vi "Normalize String.vi"(0 "String":string) -> (2 "Normalized String":string)   [LabVIEW 2013, in "JUnit XML.lvlib"]
doc: "Normalizes a string accordign to the XML specification."
uses:
  JUnit XML.lvlib
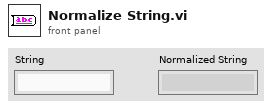
[diagram p1: front panel]
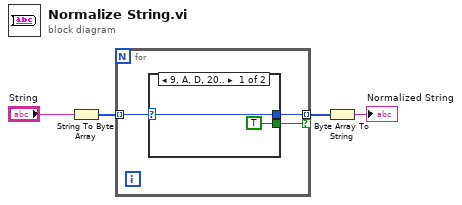
[diagram p0: block diagram]
diagram:
  n1 = String To Byte Array(string="String") -> (unsigned byte array=w3:u8[])
  n2 = for {
    tunnel: w3 -> [w7] mode=indexing
    tunnel: [w6] -> w2 mode=indexing if=w5
    n3 = case shown="9, A, D, 20.." w7 {
      selector: w7 -> [w8 _]
      tunnel: [w8 _] -> w6
      tunnel: [TRUE _] -> w5
      frame 9, 10, 13, 32.. {
      }
      frame Default {
      }
    }
  }
  n4 = Byte Array To String(unsigned byte array=w2) -> (string=→"Normalized String":string)
